vi "AccInputScale.vi"(0 "EtherCATSignal":i32, 5 "ELM3604MaxBits":i32, 7 "ELM3604MaxVolts":dbl, 9 "Acc Offset ((m/s2))":dbl, 11 "AccScale ((m/s2)/V)":dbl) -> (4 "Acc (m/s2)":dbl)   [LabVIEW 2018]
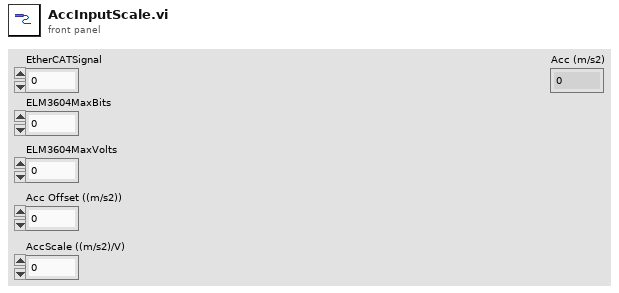
[diagram p1: front panel]
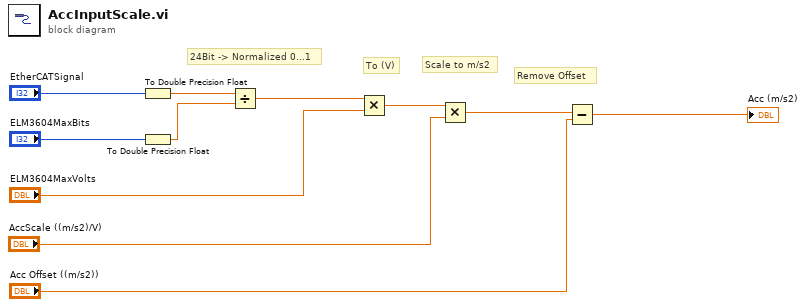
[diagram p0: block diagram]
diagram:
  # "Scale to m/s2"
  # "Remove Offset"
  # "24Bit -> Normalized 0...1"
  # "To (V)"
  n1 = To Double Precision Float(number="EtherCATSignal") -> (double precision float=w11:dbl)
  n2 = To Double Precision Float(number="ELM3604MaxBits") -> (double precision float=w9:dbl)
  n3 = Divide(x=w11, y=w9) -> (x/y=w10:dbl)
  n4 = Multiply(x=w10, y="ELM3604MaxVolts") -> (x*y=w4:dbl)
  n5 = Multiply(x=w4, y="AccScale ((m/s2)/V)") -> (x*y=w3:dbl)
  n6 = Subtract(x=w3, y="Acc Offset ((m/s2))") -> (x-y=→"Acc (m/s2)":dbl)
